vi "WS1021 Multi DUT Generate Header Ver1.5.vi"(0 "Reg 3":string[](array[string]), 1 "VPI Name":string[](array[string]), 5 "Reg 2":string[](array[string]), 11 "Error In":errorcluster) -> (4 "Header":string[](array[string]), 15 "Error Out":errorcluster)   [LabVIEW 2017]
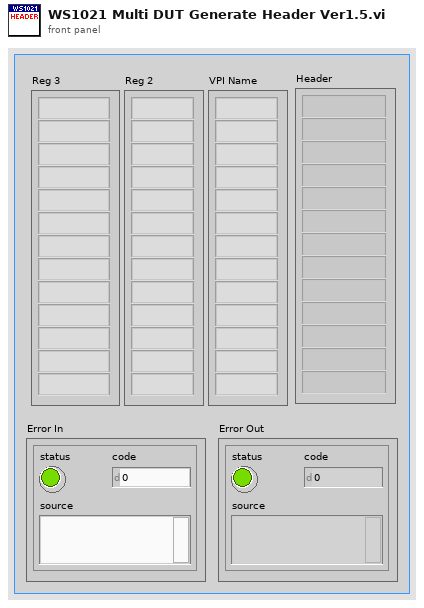
[diagram p1: front panel]
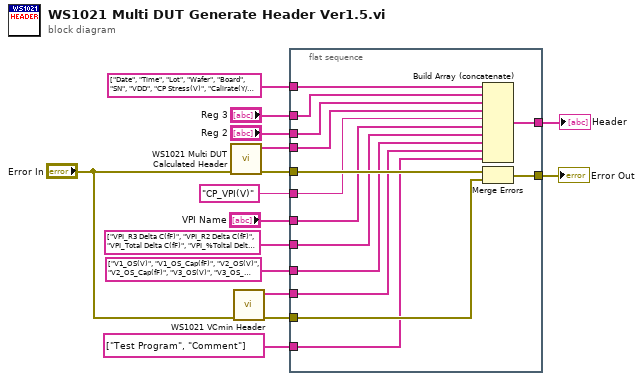
[diagram p0: block diagram]
diagram:
  n1 = call "WS1021 Multi DUT Calculated Header.vi"("Error In"="Error In") -> ("Error Out"=w9:errorcluster, "Name Calculated Header"=w8:string[])  [unwired: 9 in]
  n2 = call "WS1021 VCmin Header.vi"("Error In"="Error In") -> ("Error Out"=w4:errorcluster, "VCmin CS Header"=w3:string[])  [unwired: 9 in]
  n3 = flat-sequence {
    tunnel: w9 -> [w24]
    tunnel: "Reg 3" -> [w28]
    tunnel: "Reg 2" -> [w27]
    tunnel: string[] ["Date", "Time", "Lot", "Wafer", "Board", "SN", "VDD", "CP Stress(V)", "Calirate(Y/N)", "HS CHK(P/F)", "Freq(KHz)", "AC Mag(V)", "AC Freq(Hz)", "Set Temp_C", "Meas_Temp_C", "Meas_RH(%)", "Die X", "Die Y", "DCV(V)", "Stress Beams", "Duty Cycle(%)", "Delay Setting(us)", "Stress(Min/Num)", "Idd Stdby(uA)", "CN(fF)", "Cmin(fF)", "Idd ALL ON(uA)", "Cmax(fF)", "Idd ALL OFF(uA)", "Cmin2(fF)"] -> [w29]
    tunnel: [w22] -> w12
    tunnel: [w26] -> w11
    tunnel: "VPI Name" -> [w17]
    tunnel: w8 -> [w25]
    tunnel: string[] ["VPI_R3 Delta C(fF)", "VPI_R2 Delta C(fF)", "VPI_Total Delta C(fF)", "VPI_%Toltal Delta C"] -> [w18]
    tunnel: string[] ["V1_OS(V)", "V1_OS_Cap(fF)", "V2_OS(V)", "V2_OS_Cap(fF)", "V3_OS(V)", "V3_OS_Cap(fF)"] -> [w19]
    tunnel: w4 -> [w23]
    tunnel: w3 -> [w20]
    tunnel: string[] ["Test Program", "Comment"] -> [w21]
    tunnel: "CP_VPI(V)" -> [w16]
    frame #0 {
      n4 = Build Array (concatenate)(w29, w28, w27, w25, w16, w17, w18, w19, w20, w21) -> (w26:string[])
      n5 = Merge Errors(w24, w23) -> (w22:errorcluster)
    }
  }
  "Error Out" <- w12
  "Header" <- w11
